vi "usesPKCEWorkflow.vi"(8 "error in (no error)":errorcluster, 11 "Oauth2 in":refnum<class "Oauth2.lvclass">) -> (0 "error out":errorcluster, 2 "PKCE?":bool, 3 "Oauth2 out":refnum<class "Oauth2.lvclass">)   [LabVIEW 2020, in "Oauth2.lvclass"]
uses:
  Oauth2.lvclass
  Oauth2.lvclass/Oauth2.ctl
  OAuthToken/OAuthAccessToken.lvclass
  OAuthToken/OAuth2 Token Element -- enum.ctl
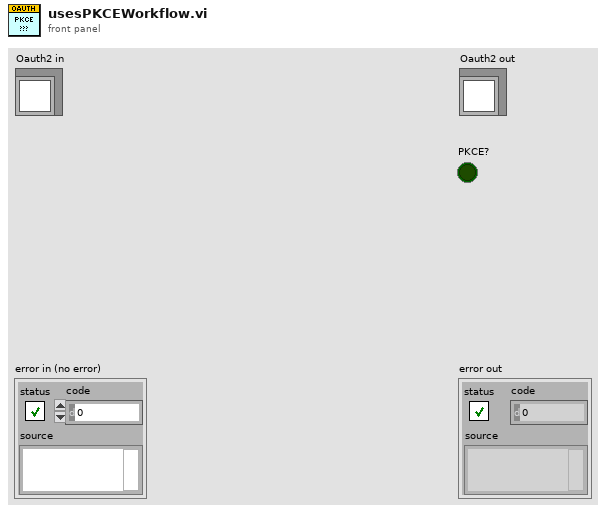
[diagram p1: front panel]
types:
  T1 = typedef "OAuthAccessToken.lvclass/OAuth2 Token Element -- enum.ctl" = enum16{"client_id", "client_secret", "response_type", "scope", "redirect_uri", "error", "error_description", "error_uri", "grant_type", "code", "access_token", "token_type", "expires_in", "username", "password", "refresh_token", "code_challenge", "code_challenge_method", "reverse_proxy_uri", "endpoint element"}
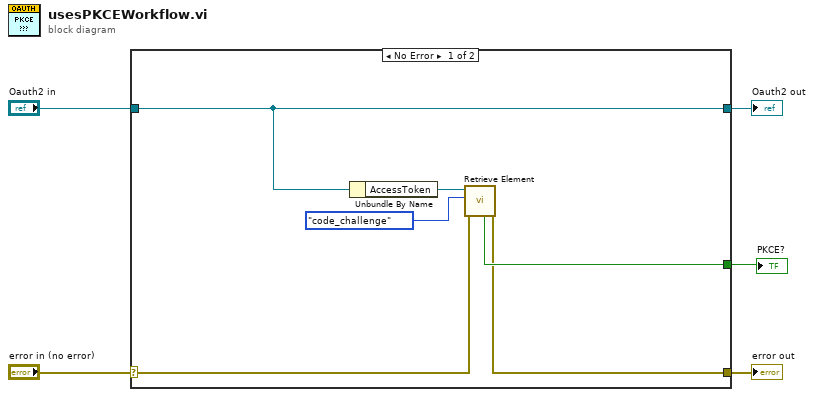
[diagram p0: block diagram]
diagram:
  n1 = case shown="No Error" "error in (no error)" {
    selector: "error in (no error)" -> [w7 w13]
    tunnel: [w6 w13] -> w4
    tunnel: [w9 w12] -> w2
    tunnel: "Oauth2 in" -> [w9 w12]
    tunnel: [w8 _] -> w1
    frame No Error {
      n2 = Unbundle By Name(w9) -> ("AccessToken"=w11:refnum<class "OAuthAccessToken.lvclass">)
      n3 = call "Retrieve Element.vi"("error in (no error)"=w7, "Token element"=OAuth2_Token_Element_--_enum."code_challenge", "OAuthAccessToken in"=w11) -> ("error out"=w6:errorcluster, "element found"=w8:bool)  [unwired: 4 in, 3 out]
    }
    frame Error {
    }
  }
  "error out" <- w4
  "Oauth2 out" <- w2
  "PKCE?" <- w1
